vi "Edgertronic-GET_cmd.vi"(3 "error in (no error)":errorcluster, 4 "Posted Content":string="/history/minutehistory.csv?MTU=2&COUNT=1440", 5 "URL":string="192.168.1.2", 6 "Type":enum16{"GET", "POST"}(ring)) -> (0 "error out":errorcluster={"status"=TRUE, "code"=1, "source"="TCP Close Connection in GrabInfoFromWeb.vi"}, 1 "data":string, 2 "Connection Info":string)   [LabVIEW 2015]
uses:
  <vilib>/httpClient/POSTBuffer.vi
  <vilib>/httpClient/LabVIEWHTTPClient.lvlib
panel:
  out "What was sent":string
  out "retrieve time":dbl=3.001
  out "read":i32
  # "http://www.myipaddress.com/show-my-ip-address/"
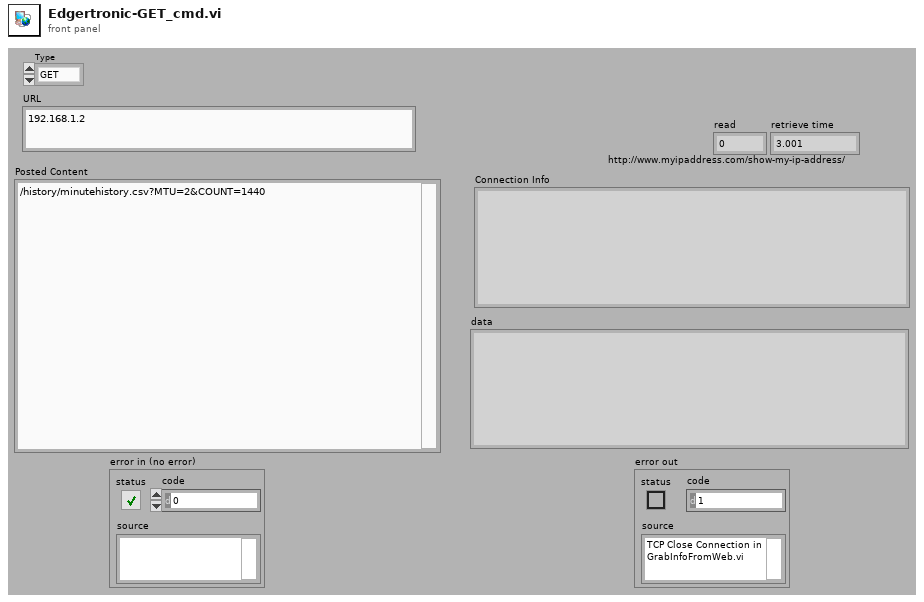
[diagram p1: front panel]
types:
  T1 = typedef "LabVIEWHTTPClient.lvlib/ClientHandle.ctl" = refnum<k1>
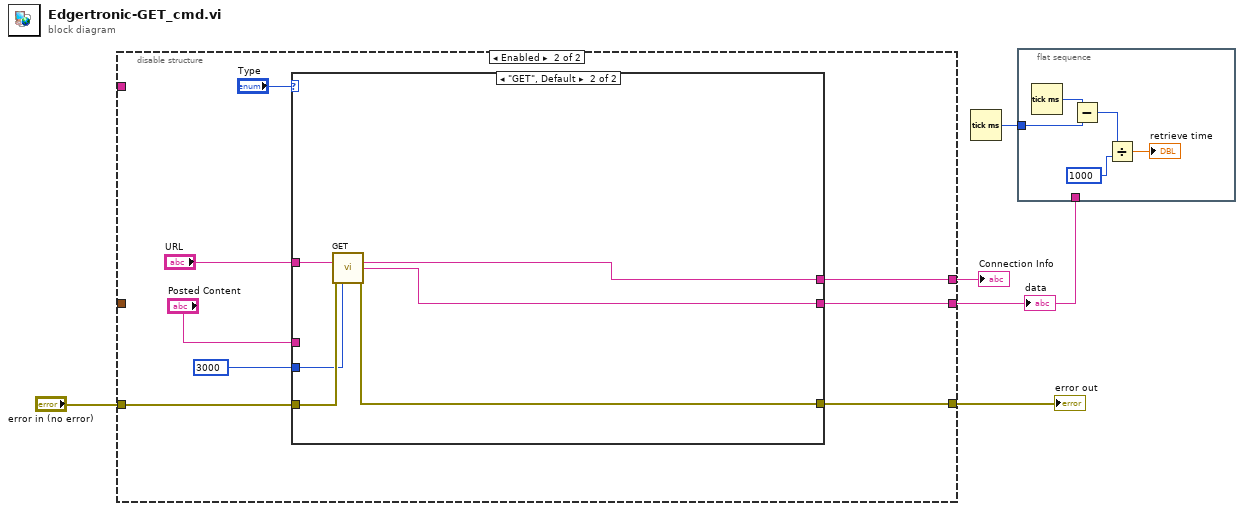
[diagram p0: block diagram]
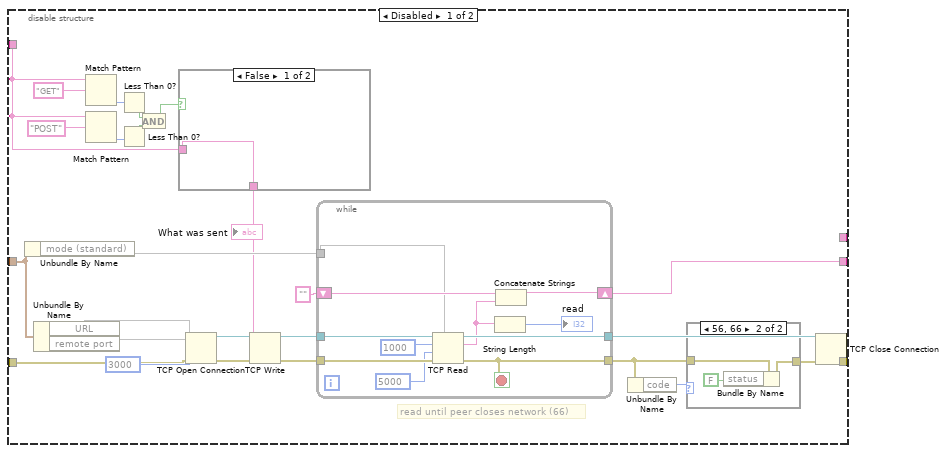
[diagram p2: hidden frame]
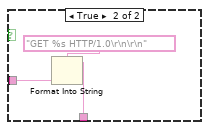
[diagram p3: hidden frame]
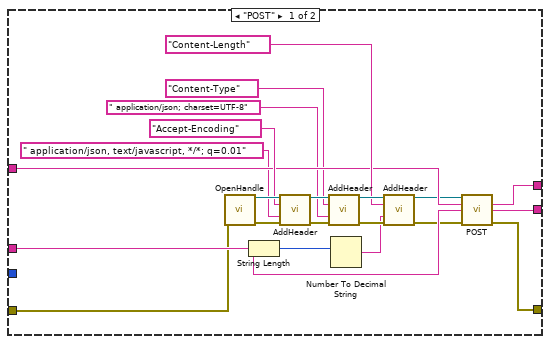
[diagram p5: hidden frame]
diagram:
  n1 = disable-structure shown="Enabled" {
    disable-tunnel: [w24 w57] -> w5
    disable-tunnel: _ -> [w21 _]
    disable-tunnel: [w16 w53] -> w1
    disable-tunnel: "error in (no error)" -> [w15 w58]
    disable-tunnel: _ -> [w12 _]
    disable-tunnel: [_ w51] -> w2
    frame Disabled {
      # "read until peer closes network (66)"
      n2 = Unbundle By Name(w21) -> ("mode (standard)"=w20)
      n3 = Unbundle By Name(w21) -> ("URL"=w23, "remote port"=w22)
      n4 = Match Pattern(string=w12, regular expression="GET") -> (offset past match=w11:i32)  [unwired: 1 in, 3 out]
      n5 = Match Pattern(string=w12, regular expression="POST") -> (offset past match=w10:i32)  [unwired: 1 in, 3 out]
      n6 = Less Than 0?(x=w11) -> (x < 0?=w9:bool)
      n7 = Less Than 0?(x=w10) -> (x < 0?=w8:bool)
      n8 = And(x=w9, y=w8) -> (x .and. y?=w7:bool)
      n9 = case shown="False" w7 {
        tunnel: [w32 w34] -> w6
        tunnel: w12 -> [w32 w33]
        frame False {
        }
        frame True {
          n10 = Format Into String(format string="GET %s HTTP/1.0\r\n\r\n" ("GET Cmd"), w33) -> (resulting string=w34:string)  [unwired: 2 in, 1 out]
        }
      }
      "What was sent" <- w6
      n11 = TCP Open Connection(address=w23, remote port or service name=w22, timeout ms (60000)=3000, error in (no error)=w15) -> (connection ID=w26:refnum<k5>, error out=w25:errorcluster)  [unwired: 1 in]
      n12 = TCP Write(connection ID=w26, data in=w6, error in (no error)=w25) -> (connection ID out=w28:refnum<k5>, error out=w27:errorcluster)  [unwired: 1 in, 1 out]
      n13 = while {
        tunnel: w27 -> [w50]
        tunnel: w28 -> [w49]
        tunnel: [w40] -> w17
        tunnel: [w48] -> w29
        shift-right: [w43] -> w16
        shift-left: "" -> [w44]
        tunnel: w20 -> [w41]
        stop <- w40 stop-if-true
        n14 = TCP Read(connection ID=w49, bytes to read=1000, error in (no error)=w50, 7:w41, 9:5000 ("timeout ms (25000)")) -> (connection ID out=w48:refnum<k5>, data out=w42:string, error out=w40:errorcluster)
        n15 = String Length(string=w42) -> (length=→"read":i32)
        n16 = Concatenate Strings(w44, w42) -> (w43:string)
      }
      n17 = Unbundle By Name(w17) -> ("code"=w19:i32)
      n18 = case shown="56, 66" w19 {
        tunnel: [w36 w38] -> w18
        tunnel: w17 -> [w36 w39]
        frame Default {
        }
        frame 56, 66 {
          n19 = Bundle By Name(cluster=w39, "status"=FALSE) -> (w38:errorcluster)
        }
      }
      n20 = TCP Close Connection(connection ID=w29, error in (no error)=w18) -> (error out=w24:errorcluster)  [unwired: 1 in, 1 out]
    }
    frame Enabled {
      n21 = case shown="\"GET\", Default" "Type" {
        tunnel: w58 -> [w68 w85]
        tunnel: [w63 w84] -> w57
        tunnel: 3000 ("timeout (10000)") -> [_ w83]
        tunnel: "URL" -> [w74 w82]
        tunnel: [w62 w81] -> w53
        tunnel: "Posted Content" -> [w73 _]
        tunnel: [w59 w80] -> w51
        frame "POST" {
          n22 = call <vilib>:"OpenHandle.vi"("error in (no error)"=w68) -> ("client handle out"=w79:T1, "error out"=w67:errorcluster)  [unwired: 13 in]
          n23 = String Length(string=w73) -> (length=w72:i32)
          n24 = call <vilib>:"AddHeader.vi"("client handle"=w79, "header"="Accept-Encoding", "value"=" application/json, text/javascript, */*; q=0.01", "error in (no error)"=w67) -> ("client handle out"=w77:T1, "error out"=w66:errorcluster)  [unwired: 10 in]
          n25 = call <vilib>:"AddHeader.vi"("client handle"=w77, "header"="Content-Type", "value"=" application/json; charset=UTF-8", "error in (no error)"=w66) -> ("client handle out"=w76:T1, "error out"=w65:errorcluster)  [unwired: 10 in]
          n26 = Number To Decimal String(number=w72) -> (decimal integer string=w61:string)  [unwired: 1 in]
          n27 = call <vilib>:"AddHeader.vi"("client handle"=w76, "header"="Content-Length", "value"=w61, "error in (no error)"=w65) -> ("client handle out"=w60:T1, "error out"=w64:errorcluster)  [unwired: 10 in]
          n28 = call-poly <vilib>:"POST.vi"("client handle"=w60, "url"=w74, "buffer"=w73, "error in (no error)"=w64) -> ("headers"=w59:string, "body"=w62:string, "error out"=w63:errorcluster)  [unwired: 8 in, 1 out]
        }
        frame "GET", Default {
          n29 = call <vilib>:"GET.vi"("url"=w82, "error in (no error)"=w85, "timeout (10000)"=w83) -> ("headers"=w80:string, "body"=w81:string, "error out"=w84:errorcluster)  [unwired: 9 in, 1 out]
        }
      }
    }
  }
  "error out" <- w5
  "data" <- w1
  "Connection Info" <- w2
  n30 = Tick Count (ms)() -> (millisecond timer value=w3:u32)
  n31 = flat-sequence {
    tunnel: w3 -> [w86]
    tunnel: w1 -> [_]
    frame #0 {
      n32 = Tick Count (ms)() -> (millisecond timer value=w87:u32)
      n33 = Subtract(x=w87, y=w86) -> (x-y=w90:u32)
      n34 = Divide(x=w90, y=1000 ("timeout ms (60000)")) -> (x/y=→"retrieve time":dbl)
    }
  }
